vi "클러벌변수01.vi"() -> ()   [LabVIEW 2014]
panel:
  in  "정지":bool
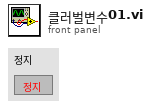
[diagram p1: front panel]
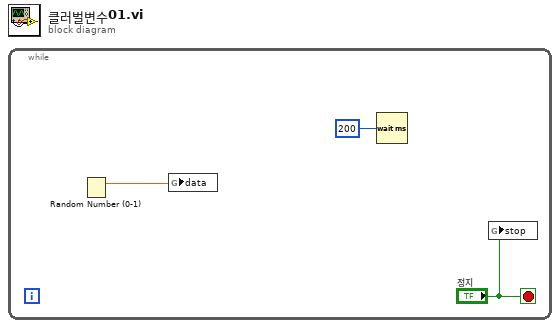
[diagram p0: block diagram]
diagram:
  n1 = while {
    stop <- "정지" stop-if-true
    n2 = Random Number (0-1)() -> (number: 0 to 1=w1:dbl)
    n3 = global write "my글로벌.vi" "data"(w1) -> ()
    n4 = Wait (ms)(milliseconds to wait=u32 200 ("대기 시간(ms)")) -> ()  [unwired: 1 out]
    n5 = global write "my글로벌.vi" "stop"("정지") -> ()
  }
